vi "promień_krzywizny.vi"(3 "e^2":ext, 4 "a":ext, 5 "fi[rad]":ext) -> (1 "Promien krzywizny południka":ext)   [LabVIEW 2015, in "Biblioteka moduł map v3.lvlib" / "Konwersja wsp.lvlib" / "UTM.lvlib"]
uses:
  UTM.lvlib
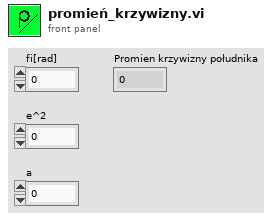
[diagram p1: front panel]
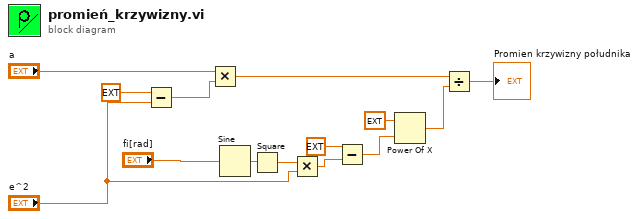
[diagram p0: block diagram]
diagram:
  n1 = Subtract(x=ext 1.0, y="e^2") -> (x-y=w2:ext)
  n2 = Multiply(x="a", y=w2) -> (x*y=w4:ext)
  n3 = Sine(x="fi[rad]") -> (sin(x)=w6:ext)
  n4 = Square(x=w6) -> (x^2=w7:ext)
  n5 = Multiply(x=w7, y="e^2") -> (x*y=w9:ext)
  n6 = Subtract(x=ext 1.0, y=w9) -> (x-y=w11:ext)
  n7 = Power Of X(1:w11, 2:ext 1.5 ("y")) -> (0:w13:ext)
  n8 = Divide(x=w4, y=w13) -> (x/y=→"Promien krzywizny południka":ext)
